vi "Set Object to Variant.vi"(8 "error in (no error)":errorcluster, 10 "Object":refnum<class>, 11 "LabVIEW Class Path":path) -> (0 "error out":errorcluster)   [LabVIEW 2016, in "SLL Class.lvlib"]
doc: "Store the Class Object in the Variant LUT."
uses:
  SLL Class.lvlib
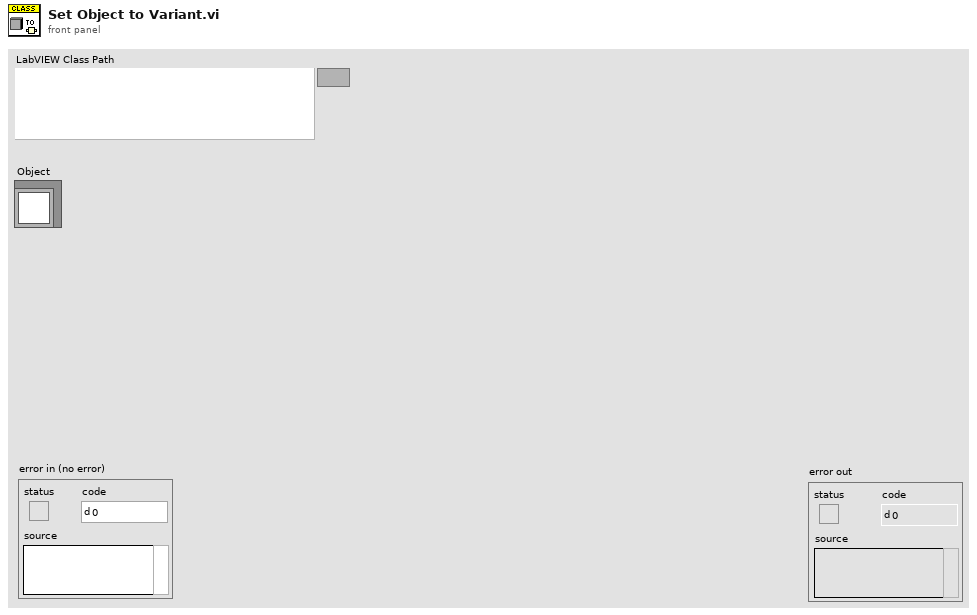
[diagram p1: front panel]
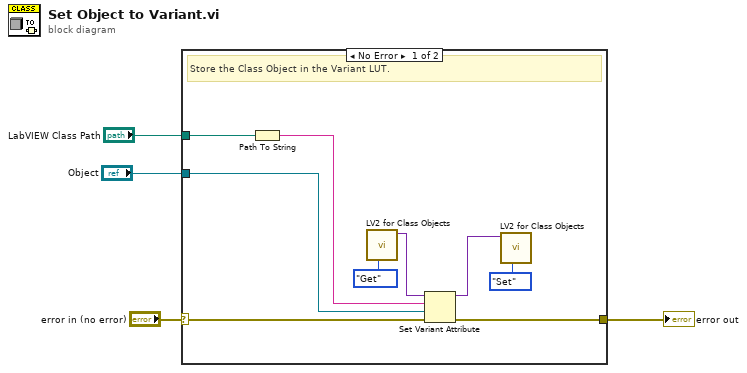
[diagram p0: block diagram]
diagram:
  n1 = case shown="No Error" "error in (no error)" {
    selector: "error in (no error)" -> [w12 w14]
    tunnel: "LabVIEW Class Path" -> [w11 _]
    tunnel: [w8 w14] -> w2
    tunnel: "Object" -> [w7 _]
    frame No Error {
      # "Store the Class Object in the Variant LUT."
      n2 = Path To String(path=w11) -> (string=w10:string)
      n3 = call "LV2 for Class Objects.vi"("Command"=enum16{"Get", "Set"}."Get") -> ("Variant Out"=w9:variant)  [unwired: 10 in]
      n4 = Set Variant Attribute(Variant=w9, name=w10, value=w7, error in=w12) -> (Variant out=w5:variant, error out=w8:errorcluster)  [unwired: 1 out]
      n5 = call "LV2 for Class Objects.vi"("Command"=enum16{"Get", "Set"}."Set", "Variant In"=w5) -> ()  [unwired: 9 in, 1 out]
    }
    frame Error {
    }
  }
  "error out" <- w2
